vi "Override Saved Settings.vi"(11 "Settings in":T1) -> (3 "Settings out":T1)   [LabVIEW 2021]
doc: "This VI overrides or resets settings that cannot be guaranteed between application launches, like the presence of devices. During startup, the application refreshes these settings to match the live state of the system."
uses:
  Acquisition/IO API.ctl
  Acquisition/Acquisition.lvlib
  Acquisition/IO Device.ctl
  Acquisition/Channel Settings.ctl
  Interval Timer/Interval Length.ctl
  Interval Timer/Interval Timer.lvlib
  Interval Timer/Repeat Interval.ctl
  Interval Timer/Interval Token.ctl
  Acquisition/Hardware Configuration.ctl
  Logging/Logging Mode.ctl
  Logging/Logging.lvlib
  Logging/Logging Configuration.ctl
  Diagnostics/Diagnostics Configuration.ctl
  Diagnostics/Diagnostics.lvlib
  Settings/Settings.ctl
  Settings/Settings.lvlib
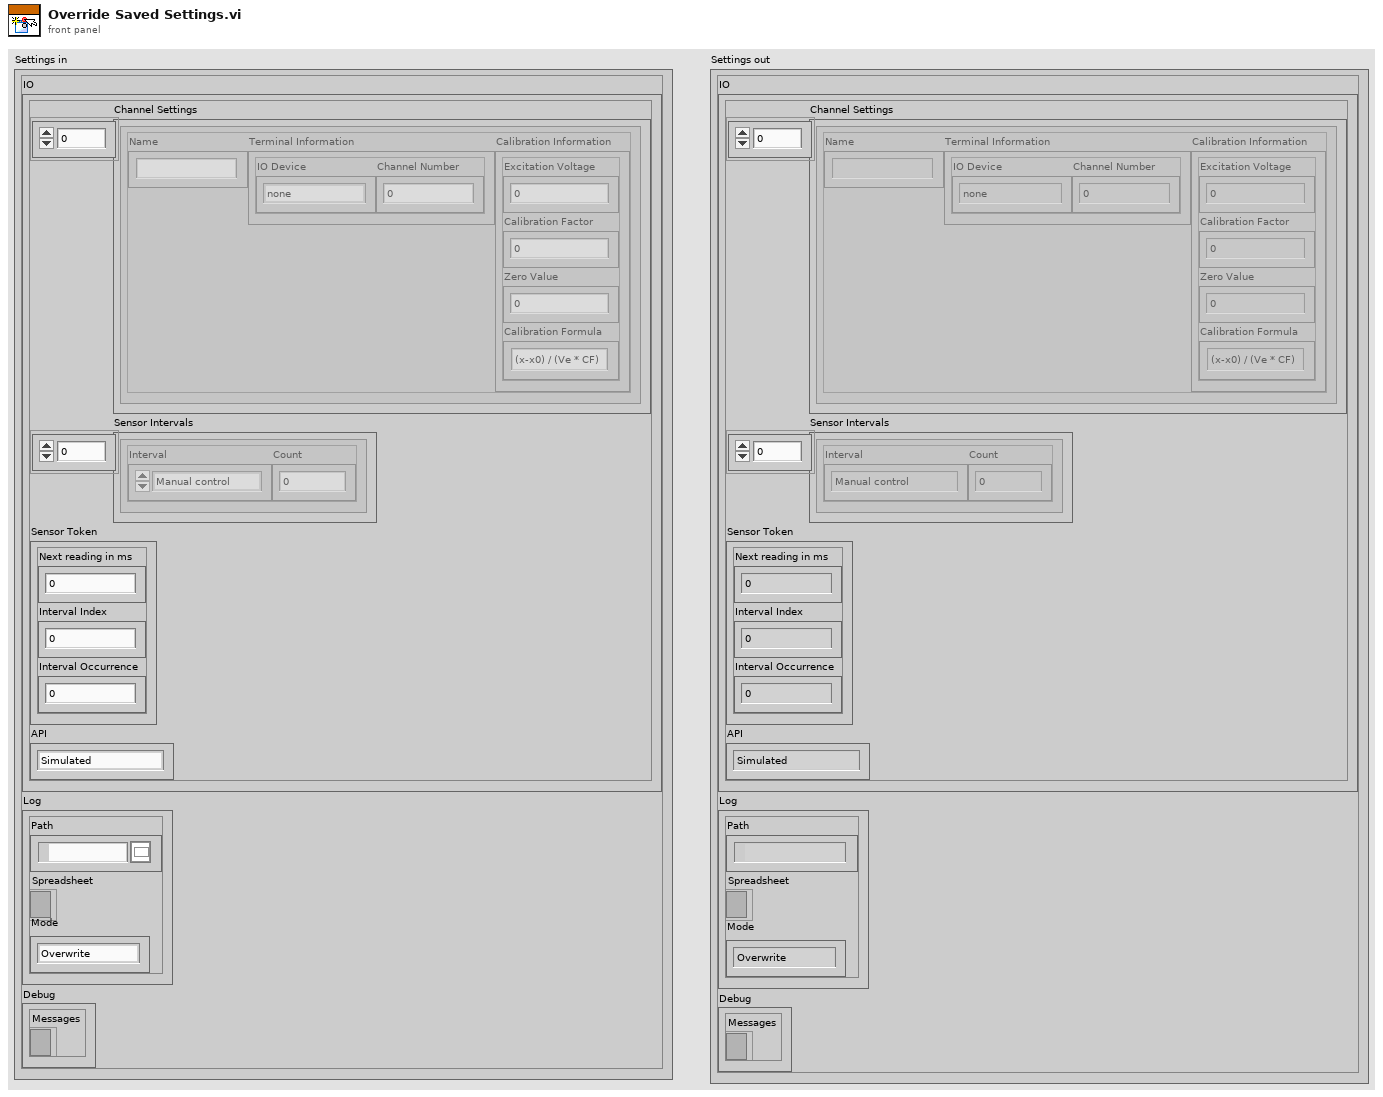
[diagram p1: front panel]
types:
  T1 = typedef "Settings.lvlib/Settings.ctl" = cluster{"IO":T2, "Log":T9, "Debug":T11}
  T2 = typedef "Acquisition.lvlib/Hardware Configuration.ctl" = cluster{"Channel Settings":T3[], "Sensor Intervals":T5[], "Sensor Token":T7, "API":T8}
  T3 = typedef "Acquisition.lvlib/Channel Settings.ctl" = cluster{"Name":string, "Terminal Information":cluster{"IO Device":T4, "Channel Number":i32}, "Calibration Information":cluster{"Excitation Voltage":dbl, "Calibration Factor":dbl, "Zero Value":dbl, "Calibration Formula":string}}
  T4 = typedef "Acquisition.lvlib/IO Device.ctl" = enum16{"none", "9219", "9401"}
  T5 = typedef "Interval Timer.lvlib/Repeat Interval.ctl" = cluster{"Interval":T6, "Count":i32}
  T6 = typedef "Interval Timer.lvlib/Interval Length.ctl" = enum16{"Manual control", "1 second", "10 seconds", "30 seconds", "60 seconds", "600 seconds", "1200 seconds", "3600 seconds"}
  T7 = typedef "Interval Timer.lvlib/Interval Token.ctl" = cluster{"Next reading in ms":u32, "Interval Index":i32, "Interval Occurrence":i32}
  T8 = typedef "Acquisition.lvlib/IO API.ctl" = enum16{"Simulated", "DAQmx"}
  T9 = typedef "Logging.lvlib/Logging Configuration.ctl" = cluster{"Path":path, "Spreadsheet":refnum<file>, "Mode":T10}
  T10 = typedef "Logging.lvlib/Logging Mode.ctl" = enum16{"Overwrite", "Append", "Create New"}
  T11 = typedef "Diagnostics.lvlib/Diagnostics Configuration.ctl" = cluster{"Messages":refnum<file>}
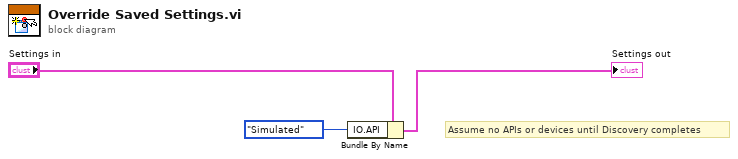
[diagram p0: block diagram]
diagram:
  # "Assume no APIs or devices until Discovery completes"
  n1 = Bundle By Name(cluster="Settings in", "IO.API"=IO_API."Simulated") -> (→"Settings out":T1)
